vi "Agilent SNA Read Averaging Factor.vi"(6 "Channel":i8=1 min=1 max=99 step=1, 7 "Agilent SNA":T1, 8 "error in (no error)":errorcluster, 11 "VISA Resource Names":T2) -> (0 "error out":errorcluster, 2 "Averaging Factor":i32, 3 "dup VISA Resource Names":T2)   [LabVIEW 2011]
doc: "This vi sets the power range. Only works on the HP 8753D."
uses:
  TypeDefs/Agilent SNA VISA.ctl
  TypeDefs/Agilent SNA Instrument Info.ctl
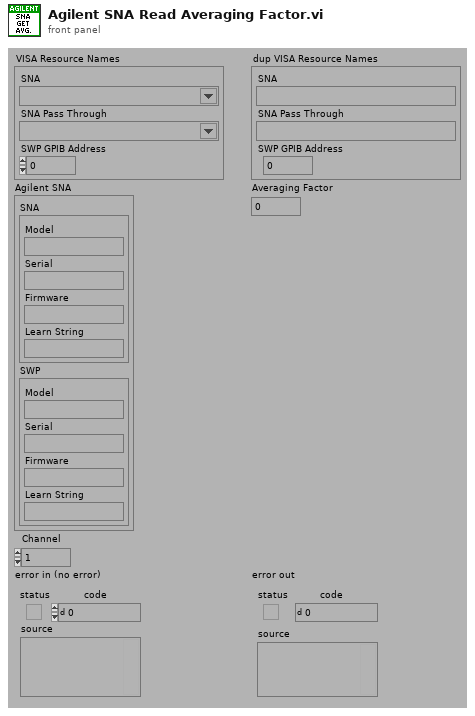
[diagram p1: front panel]
types:
  T1 = typedef "Agilent SNA Instrument Info.ctl" = cluster{"SNA":cluster{"Model":string, "Serial":string, "Firmware":string, "Learn String":string}, "SWP":cluster{"Model":string, "Serial":string, "Firmware":string, "Learn String":string}}
  T2 = typedef "Agilent SNA VISA.ctl" = cluster{"SNA":refnum<visa-resource-name>, "SNA Pass Through":refnum<visa-resource-name>, "SWP GPIB Address":i32}
  T3 = typedef "Agilent SNA Model.ctl" = enum16{"Not Supported", "8757X"}
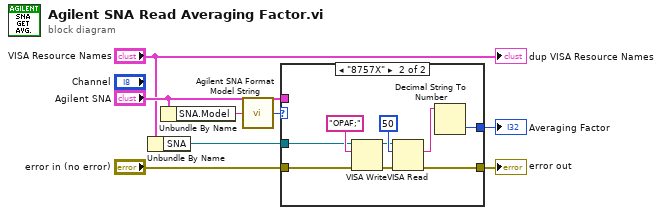
[diagram p0: block diagram]
diagram:
  n1 = Unbundle By Name("VISA Resource Names") -> ("SNA"=w1:refnum<visa-resource-name>)
  n2 = Unbundle By Name("Agilent SNA") -> ("SNA.Model"=w5:string)
  n3 = call "Agilent SNA Format Model String.vi"("Model String"=w5) -> ("Model"=w4:T3)
  n4 = case shown="\"8757X\"" w4 {
    tunnel: "error in (no error)" -> [w9 w10]
    tunnel: [_ w17] -> w7
    tunnel: [w9 w15] -> w6
    tunnel: "Agilent SNA" -> [_ _]
    tunnel: w1 -> [_ w11]
    frame "Not Supported" {
    }
    frame "8757X" {
      n5 = VISA Write(VISA resource name=w11, write buffer="OPAF;", error in (no error)=w10) -> (VISA resource name out=w13:refnum<visa-resource-name>, error out=w14:errorcluster)  [unwired: 1 out]
      n6 = VISA Read(VISA resource name=w13, byte count=u32 50, error in (no error)=w14) -> (read buffer=w18:string, error out=w15:errorcluster)  [unwired: 2 out]
      n7 = Decimal String To Number(string=w18) -> (number=w17:i32)  [unwired: 1 in, 2 out]
    }
  }
  "error out" <- w6
  "Averaging Factor" <- w7
  "dup VISA Resource Names" <- "VISA Resource Names"
